vi "PSDOM_DMG_Get Variant Value.vi"(6 "error in (no error)":errorcluster caption="错误输入（无错误）", 7 "Type String":string, 9 "Array Dimension":i32, 10 "Variant":variant) -> (1 "Cell String":string, 4 "error out":errorcluster caption="错误输出")   [LabVIEW 2013]
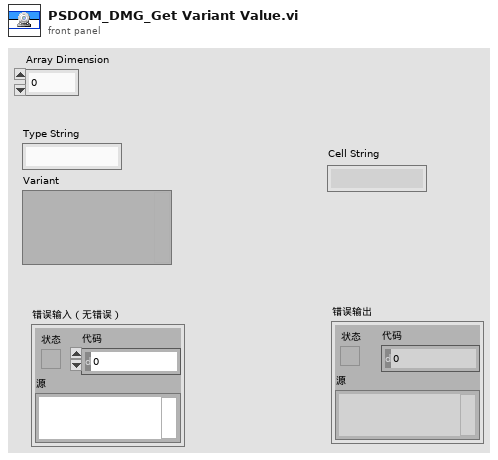
[diagram p1: front panel]
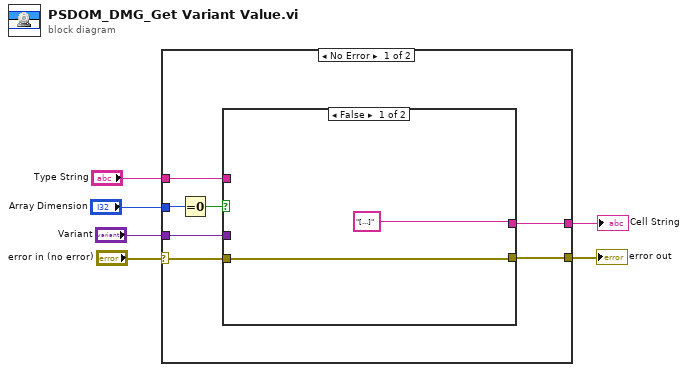
[diagram p0: block diagram]
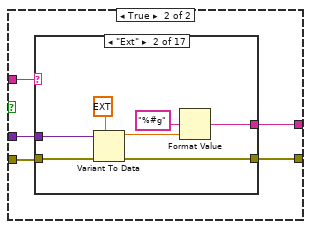
[diagram p2: hidden frame]
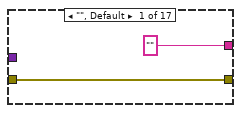
[diagram p3: hidden frame]
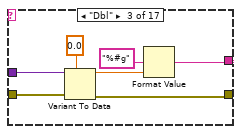
[diagram p4: hidden frame]
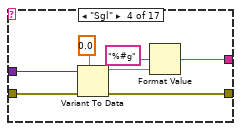
[diagram p5: hidden frame]
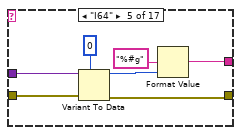
[diagram p6: hidden frame]
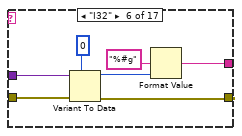
[diagram p7: hidden frame]
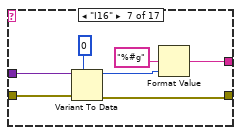
[diagram p8: hidden frame]
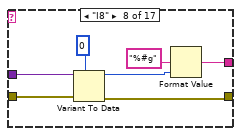
[diagram p9: hidden frame]
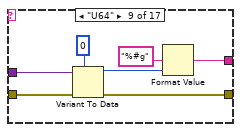
[diagram p10: hidden frame]
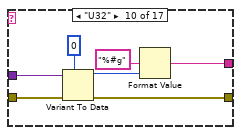
[diagram p11: hidden frame]
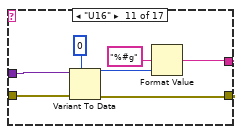
[diagram p12: hidden frame]
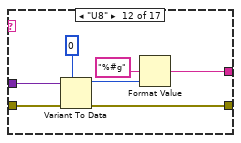
[diagram p13: hidden frame]
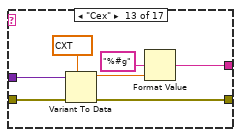
[diagram p14: hidden frame]
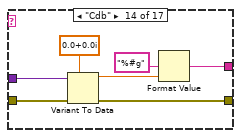
[diagram p15: hidden frame]
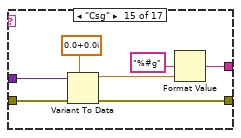
[diagram p16: hidden frame]
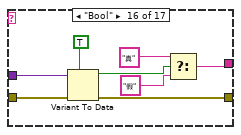
[diagram p17: hidden frame]
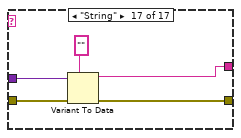
[diagram p18: hidden frame]
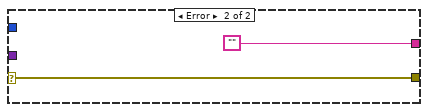
[diagram p19: hidden frame]
diagram:
  n1 = case shown="No Error" "error in (no error)" {
    selector: "error in (no error)" -> [w13 w135]
    tunnel: "Variant" -> [w12 _]
    tunnel: "Type String" -> [w11 _]
    tunnel: [w10 w135] -> w3
    tunnel: [w9 ""] -> w2
    tunnel: "Array Dimension" -> [w8 _]
    frame No Error {
      n2 = Equal To 0?(x=w8) -> (x = 0?=w7:bool)
      n3 = case shown="False" w7 {
        tunnel: w13 -> [w15 w20]
        tunnel: w12 -> [_ w19]
        tunnel: w11 -> [_ w18]
        tunnel: [w15 w17] -> w10
        tunnel: ["[...]" w16] -> w9
        frame False {
        }
        frame True {
          n4 = case shown="\"Ext\"" w18 {
            tunnel: w20 -> [w22 w27 w34 w41 w49 w55 w63 w70 w77 w84 w90 w99 w106 w113 w120 w128 w133]
            tunnel: w19 -> [_ w29 w35 w42 w50 w57 w64 w71 w78 w85 w91 w98 w105 w112 w119 w127 w132]
            tunnel: [w22 w26 w33 w40 w47 w54 w61 w69 w75 w83 w92 w97 w103 w110 w117 w125 w130] -> w17
            tunnel: ["" ("output string") w23 w30 w37 w44 w51 w58 w65 w72 w79 w86 w93 w100 w107 w114 w121 w129] -> w16
            frame "", Default {
            }
            frame "Ext" {
              n5 = Variant To Data(error in=w27, type=ext 0.0, Variant=w29) -> (data=w24:ext, error out=w26:errorcluster)
              n6 = Format Value(format string="%#g" ("格式字符串"), value (0)=w24) -> (output string=w23:string)  [unwired: 1 in]
            }
            frame "Dbl" {
              n7 = Variant To Data(error in=w34, type=0.0, Variant=w35) -> (data=w31:dbl, error out=w33:errorcluster)
              n8 = Format Value(format string="%#g" ("格式字符串"), value (0)=w31) -> (output string=w30:string)  [unwired: 1 in]
            }
            frame "Sgl" {
              n9 = Variant To Data(error in=w41, type=sgl 0.0, Variant=w42) -> (data=w38:sgl, error out=w40:errorcluster)
              n10 = Format Value(format string="%#g" ("格式字符串"), value (0)=w38) -> (output string=w37:string)  [unwired: 1 in]
            }
            frame "I64" {
              n11 = Variant To Data(error in=w49, type=i64 0, Variant=w50) -> (data=w45:i64, error out=w47:errorcluster)
              n12 = Format Value(format string="%#g" ("格式字符串"), value (0)=w45) -> (output string=w44:string)  [unwired: 1 in]
            }
            frame "I32" {
              n13 = Variant To Data(error in=w55, type=0, Variant=w57) -> (data=w52:i32, error out=w54:errorcluster)
              n14 = Format Value(format string="%#g" ("格式字符串"), value (0)=w52) -> (output string=w51:string)  [unwired: 1 in]
            }
            frame "I16" {
              n15 = Variant To Data(error in=w63, type=i16 0, Variant=w64) -> (data=w59:i16, error out=w61:errorcluster)
              n16 = Format Value(format string="%#g" ("格式字符串"), value (0)=w59) -> (output string=w58:string)  [unwired: 1 in]
            }
            frame "I8" {
              n17 = Variant To Data(error in=w70, type=i8 0, Variant=w71) -> (data=w66:i8, error out=w69:errorcluster)
              n18 = Format Value(format string="%#g" ("格式字符串"), value (0)=w66) -> (output string=w65:string)  [unwired: 1 in]
            }
            frame "U64" {
              n19 = Variant To Data(error in=w77, type=u64 0, Variant=w78) -> (data=w73:u64, error out=w75:errorcluster)
              n20 = Format Value(format string="%#g" ("格式字符串"), value (0)=w73) -> (output string=w72:string)  [unwired: 1 in]
            }
            frame "U32" {
              n21 = Variant To Data(error in=w84, type=u32 0, Variant=w85) -> (data=w80:u32, error out=w83:errorcluster)
              n22 = Format Value(format string="%#g" ("格式字符串"), value (0)=w80) -> (output string=w79:string)  [unwired: 1 in]
            }
            frame "U16" {
              n23 = Variant To Data(error in=w90, type=u16 0, Variant=w91) -> (data=w87:u16, error out=w92:errorcluster)
              n24 = Format Value(format string="%#g" ("格式字符串"), value (0)=w87) -> (output string=w86:string)  [unwired: 1 in]
            }
            frame "U8" {
              n25 = Variant To Data(error in=w99, type=u8 0, Variant=w98) -> (data=w94:u8, error out=w97:errorcluster)
              n26 = Format Value(format string="%#g" ("格式字符串"), value (0)=w94) -> (output string=w93:string)  [unwired: 1 in]
            }
            frame "Cex" {
              n27 = Variant To Data(error in=w106, type=cxt 0.0+0.0i, Variant=w105) -> (data=w101:cxt, error out=w103:errorcluster)
              n28 = Format Value(format string="%#g" ("格式字符串"), value (0)=w101) -> (output string=w100:string)  [unwired: 1 in]
            }
            frame "Cdb" {
              n29 = Variant To Data(error in=w113, type=cdb 0.0+0.0i, Variant=w112) -> (data=w108:cdb, error out=w110:errorcluster)
              n30 = Format Value(format string="%#g" ("格式字符串"), value (0)=w108) -> (output string=w107:string)  [unwired: 1 in]
            }
            frame "Csg" {
              n31 = Variant To Data(error in=w120, type=csg 0.0+0.0i, Variant=w119) -> (data=w115:csg, error out=w117:errorcluster)
              n32 = Format Value(format string="%#g" ("格式字符串"), value (0)=w115) -> (output string=w114:string)  [unwired: 1 in]
            }
            frame "Bool" {
              n33 = Variant To Data(error in=w128, type=TRUE, Variant=w127) -> (data=w124:bool, error out=w125:errorcluster)
              n34 = Select(t="真", s=w124, f="假") -> (s? t:f=w121:string)
            }
            frame "String" {
              n35 = Variant To Data(error in=w133, type="", Variant=w132) -> (data=w129:string, error out=w130:errorcluster)
            }
          }
        }
      }
    }
    frame Error {
    }
  }
  "error out" <- w3
  "Cell String" <- w2
